vi "Facebook OAuth Test.vi"() -> ()   [LabVIEW 2013]
uses:
  Oauth2/Oauth2.lvclass
  <vilib>/LabVIEW Open Source Project/OpenURI/uri/URI.lvclass
  <vilib>/httpClient/LabVIEWHTTPClient.lvlib
  Oauth2.Facebook/Oauth2.Facebook.lvclass
panel:
  out "my Profile payload":string
  out "HTTP Response Headers":string
  in  "Client Secret":string
  in  "Client ID":string
  out "Facebook Access Token":string
  out "error out":errorcluster
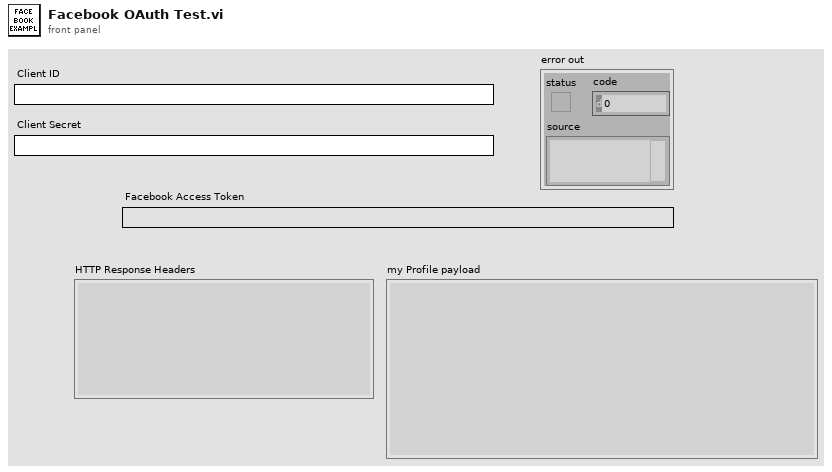
[diagram p1: front panel]
types:
  T1 = typedef "LabVIEWHTTPClient.lvlib/ClientHandle.ctl" = refnum<k1>
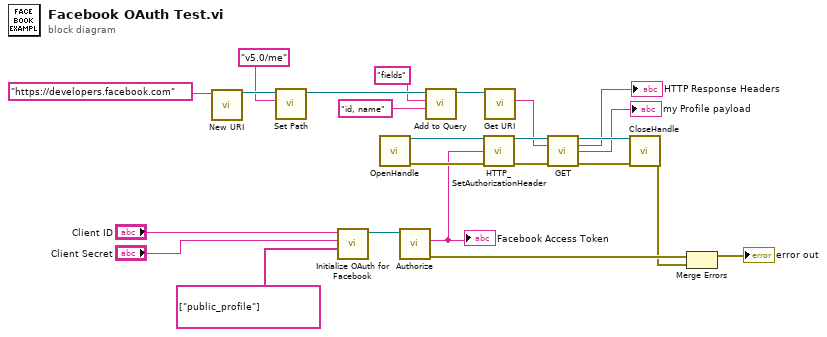
[diagram p0: block diagram]
diagram:
  n1 = call <vilib>:"New URI.vi"("URI"="https://developers.facebook.com" ("path")) -> ("URI"=w24:refnum<class "URI.lvclass">)  [unwired: 9 in, 1 out]
  n2 = call <vilib>:"Set Path.vi"("path"="v5.0/me", "URI in"=w24) -> ("URI out"=w4:refnum<class "URI.lvclass">)  [unwired: 8 in, 1 out]
  n3 = call "Initialize OAuth for Facebook.vi"("Scopes"=string[] ["public_profile"], "Client Secret"="Client Secret", "Client ID"="Client ID") -> ("Oauth2.Facebook"=w5:refnum<class "Oauth2.Facebook.lvclass">)  [unwired: 8 in]
  n4 = call <vilib>:"OpenHandle.vi"() -> ("client handle out"=w22:T1, "error out"=w21:errorcluster)  [unwired: 14 in]
  n5 = call "Authorize.vi"("Oauth2 in"=w5) -> ("error out"=w11:errorcluster, "Access Token"=w13:string)  [unwired: 8 in, 1 out]
  "Facebook Access Token" <- w13
  n6 = call <vilib>:"Add to Query.vi"("value"="id, name" ("path"), "key"="fields" ("path"), "URI in"=w4) -> ("URI out"=w3:refnum<class "URI.lvclass">)  [unwired: 7 in, 1 out]
  n7 = call "HTTP_SetAuthorizationHeader.vi"("Client Handle"=w22, "Access Token"=w13, "error in (no error)"=w21) -> ("client handle dup"=w20:T1, "error out"=w19:errorcluster)  [unwired: 11 in]
  n8 = call <vilib>:"Get URI.vi"("URI in"=w3) -> ("URI String"=w16:string)  [unwired: 8 in, 2 out]
  n9 = call <vilib>:"GET.vi"("client handle"=w20, "url"=w16, "error in (no error)"=w19) -> ("client handle out"=w18:T1, "headers"=→"HTTP Response Headers":string, "body"=→"my Profile payload":string, "error out"=w17:errorcluster)  [unwired: 9 in]
  n10 = call <vilib>:"CloseHandle.vi"("client handle"=w18, "error in (no error)"=w17) -> ("error out"=w9:errorcluster)  [unwired: 13 in]
  n11 = Merge Errors(w11, w9) -> (→"error out":errorcluster)
